vi "changeFrequence.vi"(2 "频率值":dbl=24.0 min=24.0 max=30.0 step=0.1, 3 "单片机串口":refnum<visa-resource-name>) -> (0 "字符串":string, 1 "单片机串口 2":refnum<visa-resource-name>)   [LabVIEW 2018]
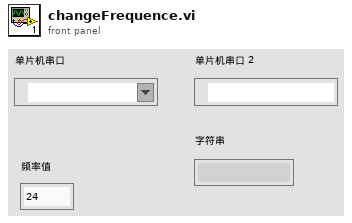
[diagram p1: front panel]
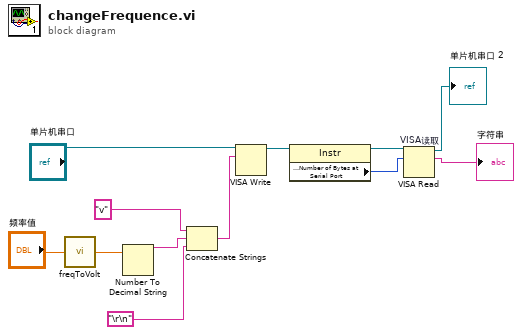
[diagram p0: block diagram]
diagram:
  n1 = call "freqToVolt.vi"("频率"="频率值") -> ("电压"=w6:dbl)
  n2 = Number To Decimal String(number=w6) -> (decimal integer string=w9:string)  [unwired: 1 in]
  n3 = Concatenate Strings("v", w9, "\r\n") -> (w7:string)
  n4 = VISA Write(VISA resource name="单片机串口", write buffer=w7) -> (VISA resource name out=w3:refnum<visa-resource-name>)  [unwired: 1 in, 2 out]
  n5 = property class="Instr"(reference=w3) -> (reference out=w2:refnum<visa-resource-name>, "Serial Settings:Number of Bytes at Serial Port"=w1:u32)  [unwired: 1 in, 1 out]
  n6 = VISA Read "VISA读取"(VISA resource name=w2, byte count=w1) -> (VISA resource name out=→"单片机串口 2":refnum<visa-resource-name>, read buffer=→"字符串":string)  [unwired: 1 in, 2 out]
